vi "Robot Velocity to LR.vi"(6 "Min Velocity":dbl, 8 "Trackwidth":dbl=30.0 format="%#_13g", 9 "Max Accel":dbl, 10 "Max Velocity":dbl, 11 "Curvature":dbl) -> (2 "r":dbl, 3 "l":dbl)   [LabVIEW 2018, in "Pure Pursuit.lvlib"]
uses:
  Pure Pursuit.lvlib
  Typedef/Path AE Action.ctl
  <vilib>/addons/control/pid/pid.llb/PID Output Rate Limiter (DBL).vi
  <vilib>/addons/control/pid/NI_PID_pid.lvlib
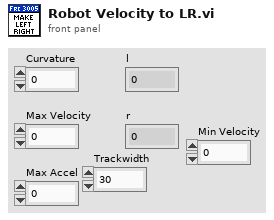
[diagram p1: front panel]
types:
  T1 = typedef "Pure Pursuit.lvlib/Path AE Action.ctl" = enum16{"Initialize", "Get Close Point", "Get Target Point", "Default", "Get Point", "Get Distance Remaining"}
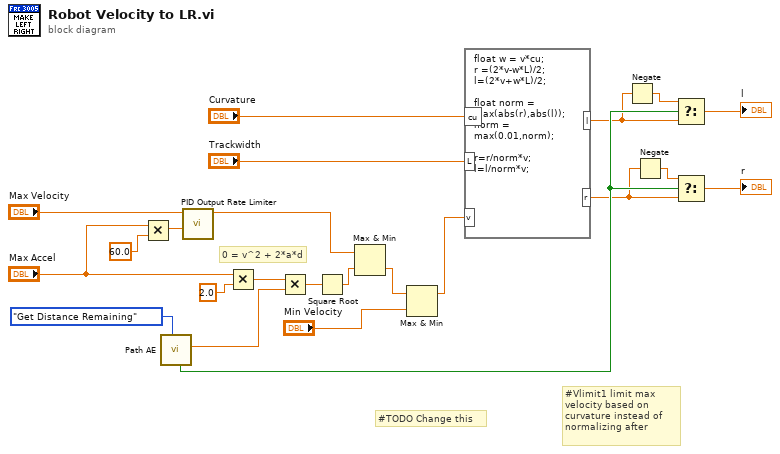
[diagram p0: block diagram]
diagram:
  # "#TODO Change this"
  # "0 = v^2 + 2*a*d"
  # "#Vlimit1 limit max velocity based on curvature instead of normalizing after"
  n1 = Multiply(x="Max Accel", y=60.0) -> (x*y=w15:dbl)
  n2 = call "Path AE.vi"("Path AE Action"=Path_AE_Action."Get Distance Remaining") -> ("Distance"=w5:dbl, "Reverse? (F)"=w10:bool)  [unwired: 5 in, 4 out]
  n3 = call-poly <vilib>:"PID Output Rate Limiter.vi"("output rate (EGU/min)"=w15, "input (controller output)"="Max Velocity") -> ("output"=w16:dbl)  [unwired: 6 in, 1 out]
  n4 = Multiply(x="Max Accel", y=2.0) -> (x*y=w18:dbl)
  n5 = Multiply(x=w18, y=w5) -> (x*y=w17:dbl)
  n6 = Square Root(x=w17) -> (sqrt(x)=w3:dbl)
  n7 = Max & Min(x=w16, y=w3) -> (min(x,y)=w2:dbl)  [unwired: 1 out]
  n8 = Max & Min(x=w2, y="Min Velocity") -> (max(x,y)=w1:dbl)  [unwired: 1 out]
  n9 = formula code="float w = v*cu;\nr =(2*v-w*L)/2;\nl=(2*v+w*L)/2;\n\nfloat norm = max(abs(r),abs(l));\nnorm = max(0.01,norm);\n\nr=r/norm*v;\nl=l/norm*v;"("L"="Trackwidth", "cu"="Curvature", "v"=w1) -> ("r"=w7:dbl, "l"=w6:dbl)
  n10 = Negate(x=w6) -> (-x=w9:dbl)
  n11 = Negate(x=w7) -> (-x=w8:dbl)
  n12 = Select(t=w9, s=w10, f=w6) -> (s? t:f=→"l":dbl)
  n13 = Select(t=w8, s=w10, f=w7) -> (s? t:f=→"r":dbl)
